vi "Edit - Data Type Library.vi"(0 "Data Type Directory":path, 5 "Data Type Library Path":path, 7 "New Data Type Name":string, 11 "error in":errorcluster) -> (4 "New Data Type Library Path":path, 6 "Old Directory to Delete":path, 15 "error out":errorcluster)   [LabVIEW 2020]
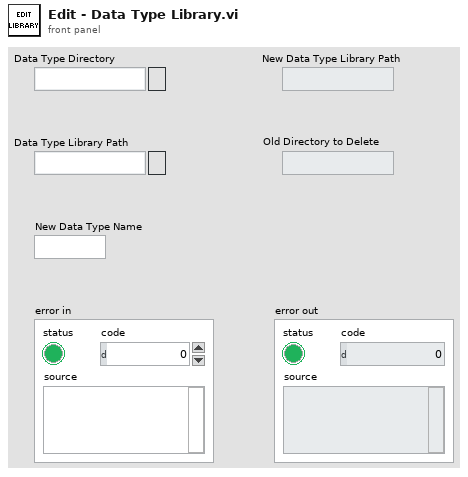
[diagram p1: front panel]
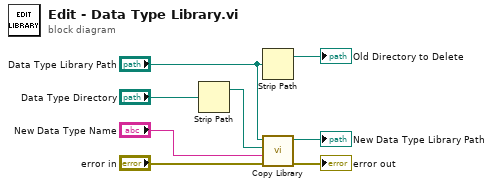
[diagram p0: block diagram]
diagram:
  n1 = Strip Path(path="Data Type Directory") -> (stripped path=w2:path)  [unwired: 1 out]
  n2 = Strip Path(path="Data Type Library Path") -> (stripped path=→"Old Directory to Delete":path)  [unwired: 1 out]
  n3 = call "Copy Library.vi"("error in (no error)"="error in", "New Name"="New Data Type Name", "Destination Directory"=w2, "Path to Library"="Data Type Library Path") -> ("error out"=→"error out":errorcluster, "New Library Path"=→"New Data Type Library Path":path)  [unwired: 6 in]
